vi "Find All Clusters.vi"(8 "Error In":errorcluster) -> (0 "Error Out":errorcluster)   [LabVIEW 2018, in "Tests.lvlib" / "Toolkit.lvlib"]
uses:
  Toolkit.lvlib
  <vilib>/addons/_JKI Toolkits/Caraya/classes/Test/Test.lvclass
  <vilib>/addons/_JKI Toolkits/Caraya/classes/Assert/Assert.lvclass
  src/Toolkit/Toolkit.lvlib
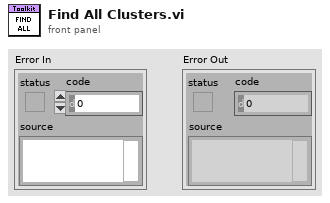
[diagram p1: front panel]
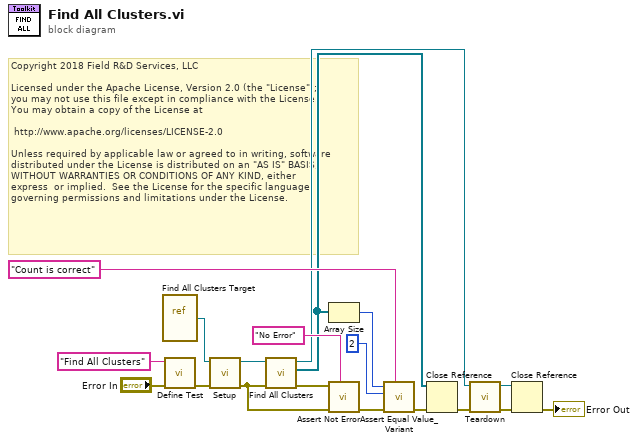
[diagram p0: block diagram]
diagram:
  # "Copyright 2018 Field R&D Services, LLC\n\nLicensed under the Apache License, Version 2.0 (the \"License\");\nyou may not use this file except in compliance with the License.\nYou may obtain a copy of the License at\n\n\thttp://www.apache.org/licenses/LICENSE-2.0\n\nUnless required by applicable law or agreed to in writing, software\ndistributed under the License is distributed on an \"AS IS\" BASIS,\nWITHOUT WARRANTIES OR CONDITIONS OF ANY KIND, either \nexpress  or implied.  See the License for the specific language \ngoverning permissions and limitations under the License."
  n1 = vi-ref "Find All Clusters Target.vi"() -> (w16:refnum<vi>)
  n2 = call <vilib>:"Define Test.vi"("error in (no error)"="Error In", "Label (VI Title)"="Find All Clusters") -> ("error out"=w17:errorcluster)  [unwired: 9 in]
  n3 = call "Setup.vi"("Error In"=w17, "VI In"=w16) -> ("Error Out"=w12:errorcluster, "VI Out"=w7:refnum<vi>)  [unwired: 8 in]
  n4 = call "Find All Clusters.vi"("Error In"=w12, "VI In"=w7) -> ("Error Out"=w13:errorcluster, "Clusters"=w1:refnum<vi>[], "VI Out"=w6:refnum<vi>)  [unwired: 7 in]
  n5 = Array Size(array=w1) -> (size(s)=w4:i32)
  n6 = call <vilib>:"Assert Not Error.vi"("Label"="No Error", "error in (no error)"=w12, "Not Error?"=w13) -> ("error out"=w5:errorcluster)  [unwired: 8 in]
  n7 = call <vilib>:"Assert Equal Value_Variant.vi"("Label"="Count is correct", "error in (no error)"=w5, "Y"=2 ("size(s)"), "X"=w4) -> ("error out"=w11:errorcluster)  [unwired: 7 in]
  n8 = Close Reference(reference=w1, error in (no error)=w11) -> (error out=w2:errorcluster)
  n9 = call "Teardown.vi"("Error In"=w2, "VI In"=w6) -> ("Error Out"=w9:errorcluster, "VI Out"=w10:refnum<vi>)  [unwired: 8 in]
  n10 = Close Reference(reference=w10, error in (no error)=w9) -> (error out=→"Error Out":errorcluster)
